vi "Main.vi"() -> ()   [LabVIEW 2016]
doc: "The myRIO Project template acquires acceleration data from the onboard accelerometer and displays the changes of acceleration values in a waveform chart."
uses:
  <vilib>/myRIO/Instrument Drivers/Onboard IO/PWM/typedefs/PWM Reference.ctl
  <vilib>/myRIO/Common/Instrument Driver Framework/Utilities/typedefs/myRIO Generic Hardware Reference.ctl
  <vilib>/myRIO/Common/Instrument Driver Framework/Utilities/typedefs/Hardware Version Enum.ctl
  <vilib>/myRIO/Common/Instrument Driver Framework/Utilities/typedefs/myRIO v1.0 Reference.ctl
  <vilib>/myRIO/Common/Instrument Driver Framework/Utilities/typedefs/Generic FPGA Reference.ctl
  <vilib>/myRIO/Common/Instrument Driver Framework/myRIO v1.0/PWM/typedefs/PWM Channels Enum.ctl
  <vilib>/myRIO/Instrument Drivers/Onboard IO/PWM/typedefs/PWM Configuration.ctl
  <vilib>/userdefined/High Color/nirio_resource_hc.ctl
  <vilib>/myRIO/Instrument Drivers/Onboard IO/AI/typedefs/AI Reference.ctl
  <vilib>/myRIO/Common/Instrument Driver Framework/myRIO v1.0/AI/typedefs/AI Channels List.ctl
  <vilib>/myRIO/Common/Instrument Driver Framework/myRIO v1.0/AI/typedefs/AI Channels Enum.ctl
  <vilib>/myRIO/Common/Instrument Driver Framework/Utilities/typedefs/Analog Scaling Constants List.ctl
  <vilib>/myRIO/Common/Instrument Driver Framework/Utilities/typedefs/Analog Scaling Constants.ctl
  <vilib>/myRIO/Instrument Drivers/Onboard IO/DIO/typedefs/DIO Reference.ctl
  <vilib>/myRIO/Common/Instrument Driver Framework/myRIO v1.0/DIO/typedefs/DIO Channels List.ctl
  <vilib>/myRIO/Common/Instrument Driver Framework/myRIO v1.0/DIO/typedefs/DIO Channels Enum.ctl
  <vilib>/myRIO/Common/Instrument Driver Framework/myRIO v1.0/PWM/vis/myRIO v1.1 Open PWM.vi
  <vilib>/myRIO/Common/Instrument Driver Framework/Utilities/vis/Is FPGA Ref Available.vi
  <vilib>/myRIO/Common/Instrument Driver Framework/myRIO v1.0/AI/vis/myRIO v1.1 Open AI.vi
  <vilib>/myRIO/Instrument Drivers/Onboard IO/AI/vis/Read.vi
  <vilib>/myRIO/Common/Instrument Driver Framework/myRIO v1.0/DIO/vis/myRIO v1.1 Open DIO.vi
  <vilib>/myRIO/Instrument Drivers/Onboard IO/DIO/vis/Read.vi
  <vilib>/myRIO/Common/Instrument Driver Framework/Utilities/vis/Validate Channels.vi
  <vilib>/myRIO/Common/Instrument Driver Framework/myRIO v1.0/PWM/vis/myRIO v1.0 Reserve PWM.vi
  <vilib>/myRIO/Common/Instrument Driver Framework/myRIO v1.0/AI/vis/myRIO v1.0 Reserve AI.vi
  <vilib>/myRIO/Common/Instrument Driver Framework/myRIO v1.0/UART/vis/myRIO v1.0 Close UART.vi
  <vilib>/myRIO/Common/Instrument Driver Framework/myRIO v1.0/DIO/vis/myRIO v1.0 Reserve DIO.vi
  <vilib>/myRIO/Common/Instrument Driver Framework/myRIO v1.0/PWM/vis/myRIO v1.0 Build MUX Configuration PWM.vi
  <vilib>/myRIO/Common/Instrument Driver Framework/myRIO v1.0/Resource Manager/vis/myRIO v1.0 Reserve Channel List.vi
  <vilib>/myRIO/Common/Instrument Driver Framework/myRIO v1.0/AI/vis/myRIO v1.0 Build MUX Configuration AI.vi
  <vilib>/myRIO/Common/Instrument Driver Framework/myRIO v1.0/DIO/vis/myRIO v1.0 Build MUX Configuration DIO.vi
  <vilib>/myRIO/Common/Instrument Driver Framework/myRIO v1.0/Resource Manager/vis/myRIO v1.0 Create Configuration List.vi
  <vilib>/myRIO/Common/Instrument Driver Framework/myRIO v1.0/Resource Manager/vis/myRIO v1.0 Reserve Channel.vi
  <vilib>/myRIO/Common/Instrument Driver Framework/myRIO v1.0/Resource Manager/vis/myRIO v1.0 Unreserve Channel.vi
  <vilib>/myRIO/Common/Instrument Driver Framework/myRIO v1.0/Resource Manager/vis/myRIO v1.0 Build Mutex Name.vi
  <vilib>/Utility/VariantDataType/GetNumericInfo.vi
  <vilib>/Utility/error.llb/Error Cluster From Error Code.vi
  <vilib>/myRIO/Common/Instrument Driver Framework/myRIO v1.0/myRIO v1.1 Open.vi
  <vilib>/myRIO/Common/Instrument Driver Framework/Utilities/vis/IO Manager.vi
  <vilib>/myRIO/Common/Instrument Driver Framework/Utilities/vis/Configuration Manager.vi
  <vilib>/myRIO/Common/Instrument Driver Framework/myRIO v1.0/Resource Manager/vis/myRIO v1.0 Configure IO.vi
  <vilib>/myRIO/Common/Instrument Driver Framework/myRIO v1.0/myRIO v1.0 Close.vi
  <vilib>/myRIO/Common/Instrument Driver Framework/myRIO v1.0/DIO/vis/myRIO v1.0 Read DIO.vi
  <vilib>/myRIO/Common/Instrument Driver Framework/myRIO v1.0/PWM/vis/myRIO v1.0 Write PWM.vi
  <vilib>/myRIO/Common/Instrument Driver Framework/Utilities/vis/FPGA Ref Manager.vi
  <vilib>/myRIO/Common/Instrument Driver Framework/myRIO v1.0/myRIO v1.0 Reset FPGA.vi
  <vilib>/myRIO/Common/Instrument Driver Framework/myRIO v1.0/IRQ/vis/myRIO v1.0 IRQ Info FGV.vi
  <vilib>/myRIO/Common/Instrument Driver Framework/myRIO v1.0/IRQ/vis/myRIO v1.0 Timer IRQ Info FGV.vi
  <vilib>/myRIO/Common/Instrument Driver Framework/myRIO v1.0/IRQ/vis/myRIO v1.0 ISR Agent.vi
  <vilib>/myRIO/Common/Instrument Driver Framework/myRIO v1.0/AI/vis/myRIO v1.0 Get Scaling Constants AI.vi
  <vilib>/myRIO/Common/Instrument Driver Framework/myRIO v1.0/AI/vis/myRIO v1.0 Read AI.vi
  <vilib>/myRIO/Instrument Drivers/Onboard IO/PWM/vis/myRIO PWM Open.xnode
  <vilib>/myRIO/Express VI/Onboard IO/DI/DI Express VI.xnode
  <vilib>/myRIO/Instrument Drivers/Onboard IO/DIO/vis/myRIO DIO Open.xnode
  <vilib>/myRIO/Express VI/Onboard IO/AI/AI Express VI.xnode
  <vilib>/myRIO/Instrument Drivers/Onboard IO/AI/vis/myRIO AI Open.xnode
  <vilib>/myRIO/Instrument Drivers/Onboard IO/DIO/DIO.lvlib
  <vilib>/myRIO/Instrument Drivers/Onboard IO/PWM/PWM.lvlib
  <vilib>/myRIO/Instrument Drivers/Utilities/Utilities.lvlib
  <vilib>/myRIO/Instrument Drivers/Onboard IO/AI/AI.lvlib
panel:
  in  "Geschwindigkeit":dbl(knob)=0.1402796355699434 scale=0.0..1.0
  in  "stop 2":bool
  in  "stop":bool
  out "output nach1/x":dbl=0.2857142857142857
  out "Gas Motor":dbl=0.31549826192348907
  out "position":dbl(knob)=0.31549826192348907 step=0.01 scale=0.2..0.4
  in  "Frequenz 2":dbl=200.0
  out "Strom 2":dbl=-149.04557758721205
  out "Wert 2":dbl=0.241699194
  out "Waveform Chart 2":dbl(graph)=-149.04557758721205
  in  "Korrektur":dbl=15.0
  out "output Array":dbl=-3.5 format="%.2f"
  out "A/DIO7 (Pin 25)":bool
  out "A/DIO6 (Pin 23)":bool
  out "A/DIO5 (Pin 21)":bool
  out "A/DIO4 (Pin 19)":bool
  out "A/DIO3 (Pin 17)":bool
  out "A/DIO2 (Pin 15)":bool
  out "A/DIO1 (Pin 13)":bool=TRUE
  out "A/DIO0 (Pin 11)":bool=TRUE
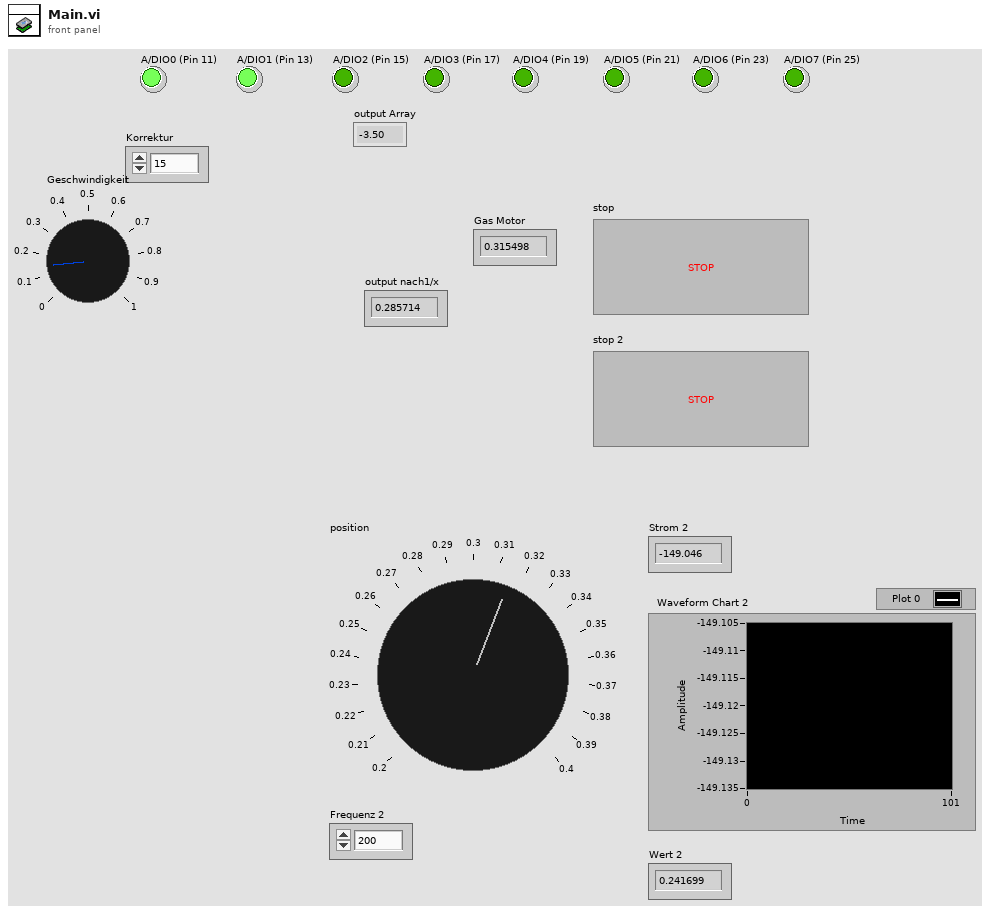
[diagram p1: front panel]
types:
  T1 = typedef "PWM.lvlib/PWM Reference.ctl" = cluster{"myRIO Reference":T2, "PWM Channels Enum":T6, "PWM Configuration":T7}
  T2 = typedef "myRIO Generic Hardware Reference.ctl" = cluster{"myRIO Model":T3, "myRIO Hardware Reference":T4}
  T3 = typedef "Hardware Version Enum.ctl" = enum16{"Unknown", "myRIO-1900", "myRIO-1950", "roboRIO", "NI ELVIS RIO CM"}
  T4 = typedef "myRIO v1.0 Reference.ctl" = cluster{"Generic FPGA Reference":T5, "Allow multiple opens":bool}
  T5 = typedef "Generic FPGA Reference.ctl" = refnum<k20>
  T6 = typedef "PWM Channels Enum.ctl" = enum16{"Not Connected", "C/PWM0", "C/PWM1", "A/PWM0", "A/PWM1", "A/PWM2", "B/PWM0", "B/PWM1", "B/PWM2", "PWM/PWM0", "PWM/PWM1", "PWM/PWM2", "PWM/PWM3", "PWM/PWM4", "PWM/PWM5", "PWM/PWM6", "PWM/PWM7", "PWM/PWM8", "PWM/PWM9"}
  T7 = typedef "PWM.lvlib/PWM Configuration.ctl" = cluster{"Frequency":dbl, "Duty Cycle":dbl}
  T8 = typedef "DIO.lvlib/DIO Reference.ctl" = cluster{"myRIO Reference":T2, "DIO Channels List":T9}
  T9 = typedef "DIO Channels List.ctl" = T10[]
  T10 = typedef "DIO Channels Enum.ctl" = enum16{"Not Connected", "C/DIO0", "C/DIO1", "C/DIO2", "C/DIO3", "C/DIO4", "C/DIO5", "C/DIO6", "C/DIO7", "A/DIO0", "A/DIO1", "A/DIO2", "A/DIO3", "A/DIO4", "A/DIO5", "A/DIO6", "A/DIO7", "A/DIO8", "A/DIO9", "A/DIO10", "A/DIO11", "A/DIO12", "A/DIO13", "A/DIO14", "A/DIO15", "B/DIO0", "B/DIO1", "B/DIO2", "B/DIO3", "B/DIO4", "B/DIO5", "B/DIO6", "B/DIO7", "B/DIO8", "B/DIO9", "B/DIO10", "B/DIO11", "B/DIO12", "B/DIO13", "B/DIO14", "B/DIO15", "LED0", "LED1", "LED2", "LED3", "Button0", "DIO/DIO0", "DIO/DIO1", "DIO/DIO2", "DIO/DIO3", "DIO/DIO4", "DIO/DIO5", "DIO/DIO6", "DIO/DIO7", "DIO/DIO8", "DIO/DIO9", "SPI/CS0", "SPI/CS1", "SPI/CS2", "SPI/CS3", "LED RADIO (Green)", "LED RADIO (Red)", "LED COMM (Green)", "LED COMM (Red)", "LED MODE (Green)", "LED MODE (Red)"}
  T11 = typedef "nirio_resource_hc.ctl" = tag
  T12 = typedef "AI.lvlib/AI Reference.ctl" = cluster{"myRIO Reference":T2, "AI Channels List":T13, "AI Scaling Constants List":T15}
  T13 = typedef "AI Channels List.ctl" = T14[]
  T14 = typedef "AI Channels Enum.ctl" = enum16{"Not Connected", "AudioIn/Left", "AudioIn/Right", "C/AI0", "C/AI1", "A/AI0", "A/AI1", "A/AI2", "A/AI3", "B/AI0", "B/AI1", "B/AI2", "B/AI3", "AI/AI0", "AI/AI1", "AI/AI2", "AI/AI3"}
  T15 = typedef "Analog Scaling Constants List.ctl" = T16[]
  T16 = typedef "Analog Scaling Constants.ctl" = cluster{"LSB Weight (Volts)":dbl, "Offset (Volts)":dbl, "Signed?":bool}
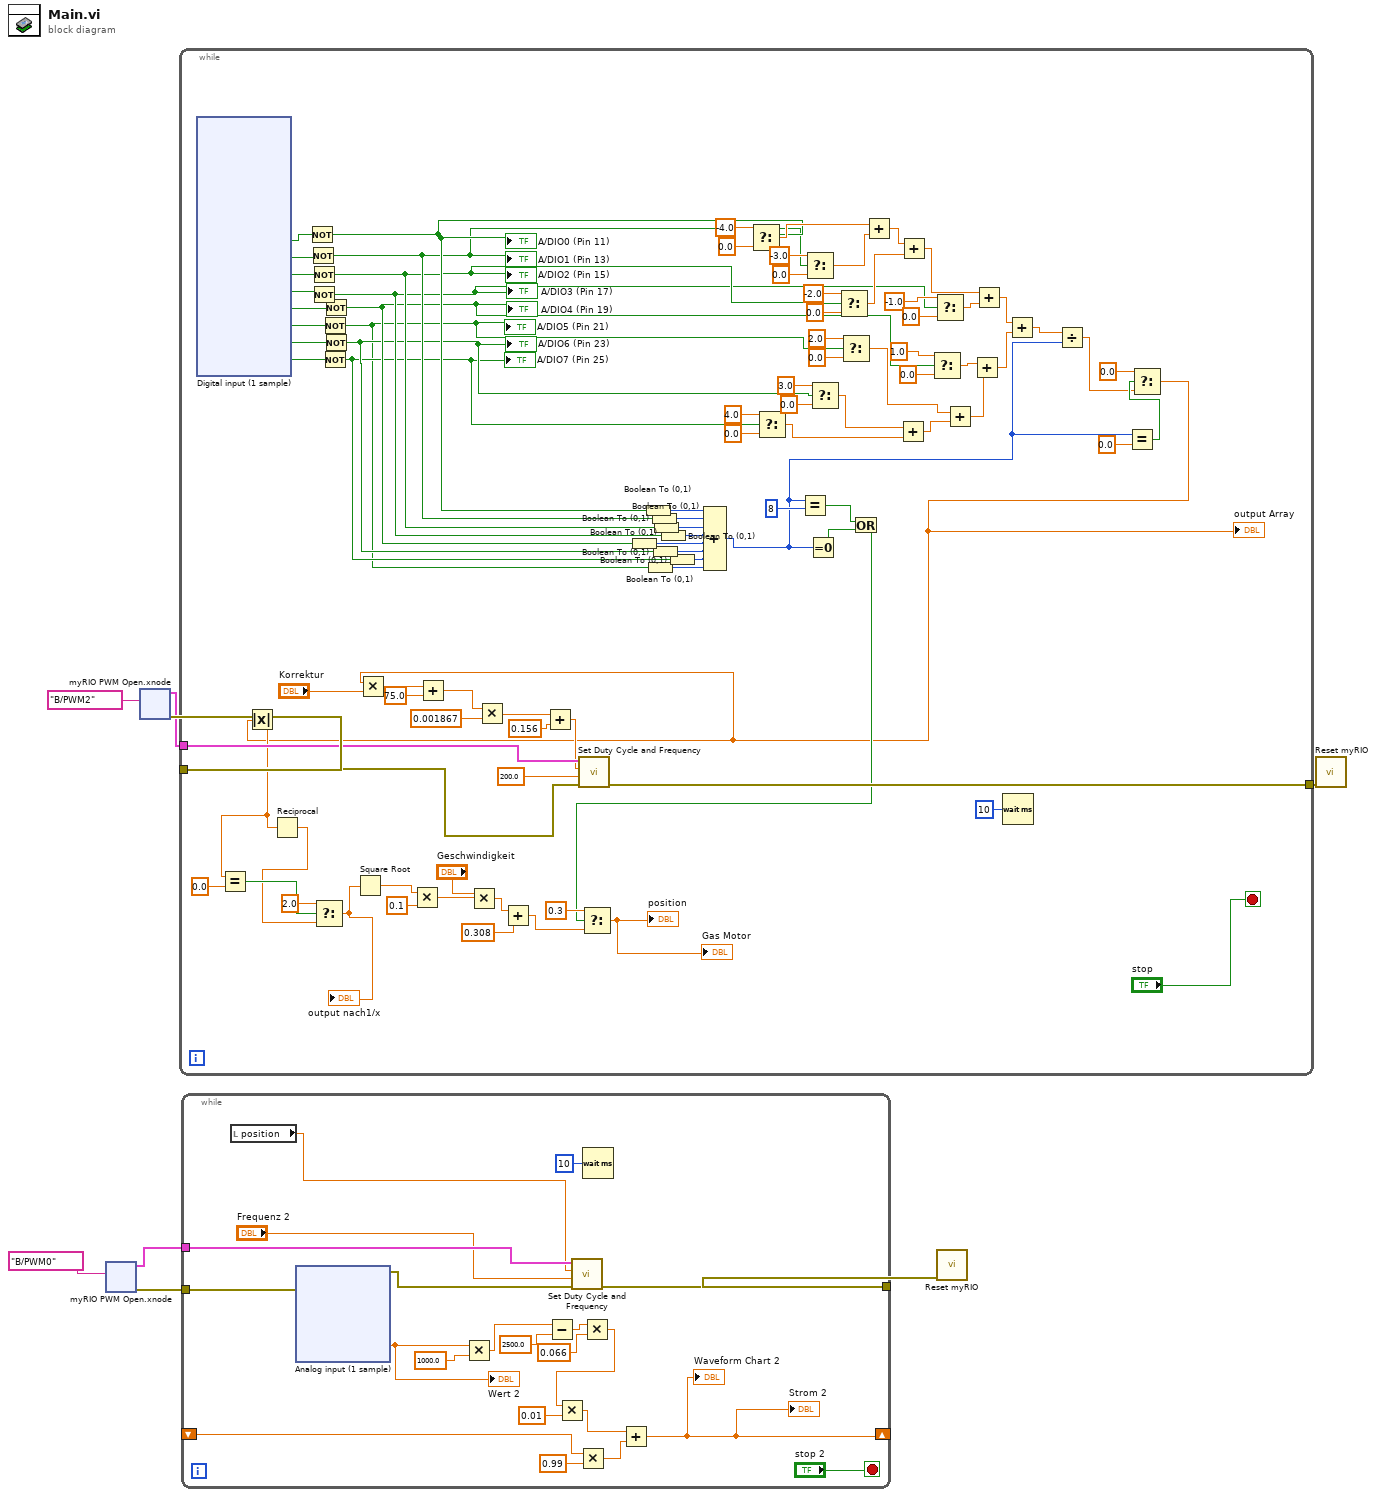
[diagram p0: block diagram]
diagram:
  n1 = xnode "myRIO PWM Open.xnode"("Channel Name"=tag "B/PWM0") -> ("error out"=w2:errorcluster, "PWM Ref Out"=w3:T1)  [unwired: 2 in]
  n2 = xnode "myRIO PWM Open.xnode"("Channel Name"=tag "B/PWM2") -> ("error out"=w7:errorcluster, "PWM Ref Out"=w6:T1)  [unwired: 2 in]
  n3 = while {
    tunnel: w7 -> [w64]
    tunnel: w6 -> [w102]
    tunnel: [w101] -> w5
    stop <- "stop" stop-if-true
    n4 = xnode "Digital input (1 sample)"() -> ("A/DIO0 (Pin 11)"=w44:bool, "A/DIO1 (Pin 13)"=w42:bool, "A/DIO2 (Pin 15)"=w40:bool, "A/DIO3 (Pin 17)"=w39:bool, "A/DIO4 (Pin 19)"=w38:bool, "A/DIO5 (Pin 21)"=w37:bool, "A/DIO6 (Pin 23)"=w36:bool, "A/DIO7 (Pin 25)"=w30:bool)  [unwired: 1 in, 1 out]
    n5 = Not(x=w44) -> (.not. x?=w43:bool)
    "A/DIO0 (Pin 11)" <- w43
    n6 = Not(x=w42) -> (.not. x?=w41:bool)
    "A/DIO1 (Pin 13)" <- w41
    n7 = Not(x=w40) -> (.not. x?=w24:bool)
    "A/DIO2 (Pin 15)" <- w24
    n8 = Not(x=w39) -> (.not. x?=w23:bool)
    "A/DIO3 (Pin 17)" <- w23
    n9 = Not(x=w37) -> (.not. x?=w19:bool)
    "A/DIO5 (Pin 21)" <- w19
    n10 = Not(x=w30) -> (.not. x?=w20:bool)
    "A/DIO7 (Pin 25)" <- w20
    n11 = Not(x=w38) -> (.not. x?=w22:bool)
    "A/DIO4 (Pin 19)" <- w22
    n12 = Not(x=w36) -> (.not. x?=w21:bool)
    "A/DIO6 (Pin 23)" <- w21
    n13 = Boolean To (0,1)(Boolean=w22) -> (0, 1=w14:i16)
    n14 = Boolean To (0,1)(Boolean=w43) -> (0, 1=w18:i16)
    n15 = Boolean To (0,1)(Boolean=w19) -> (0, 1=w11:i16)
    n16 = Boolean To (0,1)(Boolean=w41) -> (0, 1=w17:i16)
    n17 = Boolean To (0,1)(Boolean=w21) -> (0, 1=w13:i16)
    n18 = Boolean To (0,1)(Boolean=w24) -> (0, 1=w16:i16)
    n19 = Boolean To (0,1)(Boolean=w23) -> (0, 1=w15:i16)
    n20 = Boolean To (0,1)(Boolean=w20) -> (0, 1=w12:i16)
    n21 = Compound Arithmetic op=ADD(w18, w17, w16, w15, w14, w13, w12, w11) -> (w10:i16)
    n22 = Select(t=-4.0, s=w43, f=0.0) -> (s? t:f=w89:dbl)
    n23 = Select(t=4.0, s=w20, f=0.0) -> (s? t:f=w81:dbl)
    n24 = Equal?(x=w10, y=u32 8) -> (x = y?=w33:bool)
    n25 = Select(t=-3.0, s=w41, f=0.0) -> (s? t:f=w88:dbl)
    n26 = Equal To 0?(x=w10) -> (x = 0?=w35:bool)
    n27 = Select(t=3.0, s=w21, f=0.0) -> (s? t:f=w80:dbl)
    n28 = Select(t=-2.0, s=w24, f=0.0) -> (s? t:f=w86:dbl)
    n29 = Select(t=2.0, s=w19, f=0.0) -> (s? t:f=w78:dbl)
    n30 = Or(x=w33, y=w35) -> (x .or. y?=w34:bool)
    n31 = Add(x=w89, y=w88) -> (x+y=w87:dbl)
    n32 = Add(x=w80, y=w81) -> (x+y=w79:dbl)
    n33 = Add(x=w87, y=w86) -> (x+y=w83:dbl)
    n34 = Select(t=1.0, s=w22, f=0.0) -> (s? t:f=w76:dbl)
    n35 = Select(t=-1.0, s=w23, f=0.0) -> (s? t:f=w82:dbl)
    n36 = Add(x=w78, y=w79) -> (x+y=w77:dbl)
    n37 = Add(x=w76, y=w77) -> (x+y=w70:dbl)
    n38 = Add(x=w83, y=w82) -> (x+y=w71:dbl)
    n39 = Wait (ms)(milliseconds to wait=u32 10) -> ()  [unwired: 1 out]
    n40 = Add(x=w71, y=w70) -> (x+y=w69:dbl)
    n41 = Divide(x=w69, y=w10) -> (x/y=w65:dbl)
    n42 = Equal?(x=w10, y=0.0) -> (x = y?=w67:bool)
    n43 = Select(t=0.0, s=w67, f=w65) -> (s? t:f=w9:dbl)
    "output Array" <- w9
    n44 = Absolute Value(x=w9) -> (abs(x)=w48:dbl)
    n45 = Equal?(x=w48, y=0.0) -> (x = y?=w53:bool)
    n46 = Reciprocal(x=w48) -> (1/x=w49:dbl)
    n47 = Select(t=2.0, s=w53, f=w49) -> (s? t:f=w26:dbl)
    "output nach1/x" <- w26
    n48 = Square Root(x=w26) -> (sqrt(x)=w25:dbl)
    n49 = Multiply(x=w9, y="Korrektur") -> (x*y=w57:dbl)
    n50 = Multiply(x=w25, y=0.1) -> (x*y=w29:dbl)
    n51 = Add(x=w57, y=75.0) -> (x+y=w56:dbl)
    n52 = Multiply(x="Geschwindigkeit", y=w29) -> (x*y=w27:dbl)
    n53 = Multiply(x=w56, y=0.001867) -> (x*y=w61:dbl)
    n54 = Add(x=w27, y=0.308) -> (x+y=w46:dbl)
    n55 = Add(x=w61, y=0.156) -> (x+y=w59:dbl)
    n56 = call <vilib>:"Set Duty Cycle and Frequency.vi"("error in (no error)"=w64, "Frequency [Hz]"=200.0 ("y"), "Duty Cycle"=w59, "PWM Ref In"=w102) -> ("error out"=w101:errorcluster)  [unwired: 5 in, 1 out]
    n57 = Select(t=0.3, s=w34, f=w46) -> (s? t:f=→"position" →"Gas Motor":dbl)
  }
  n58 = while {
    tunnel: w2 -> [w156]
    tunnel: w3 -> [w165]
    tunnel: [w164] -> w4
    shift-right: [w147] -> _
    shift-left: _ -> [w149]
    stop <- "stop 2" stop-if-true
    n59 = local read "position"() -> (w145:dbl)
    n60 = xnode "Analog input (1 sample)"("error in (no error)"=w156) -> ("A/AI3 (Pin 9)"=w157:dbl, "error out"=w155:errorcluster)
    "Wert 2" <- w157
    n61 = Multiply(x=w157, y=1000.0) -> (x*y=w154:dbl)
    n62 = Subtract(x=w154, y=2500.0) -> (x-y=w159:dbl)
    n63 = call <vilib>:"Set Duty Cycle and Frequency.vi"("error in (no error)"=w155, "Frequency [Hz]"="Frequenz 2", "Duty Cycle"=w145, "PWM Ref In"=w165) -> ("error out"=w164:errorcluster)  [unwired: 5 in, 1 out]
    n64 = Multiply(x=w149, y=0.99) -> (x*y=w148:dbl)
    n65 = Multiply(x=w159, y=0.066) -> (x*y=w153:dbl)
    n66 = Multiply(x=w153, y=0.01) -> (x*y=w150:dbl)
    n67 = Wait (ms)(milliseconds to wait=u32 10) -> ()  [unwired: 1 out]
    n68 = Add(x=w150, y=w148) -> (x+y=w147:dbl)
    "Strom 2" <- w147
    "Waveform Chart 2" <- w147
  }
  n69 = call <vilib>:"Reset myRIO.vi"("error in (no error)"=w4) -> ()  [unwired: 10 in, 1 out]
  n70 = call <vilib>:"Reset myRIO.vi"("error in (no error)"=w5) -> ()  [unwired: 10 in, 1 out]
